vi "Actor Core.vi"(8 "error in":errorcluster, 11 "Nested in":refnum<class "Binary counter.lvclass">) -> (0 "error out":errorcluster, 3 "Actor out":refnum<class "Actor.lvclass">)   [LabVIEW 2020, in "Binary counter.lvlib" / "Binary counter.lvclass"]
doc: "(<B>Filename</B>: Actor Framework.lvlib:Actor.lvclass:Actor Core.vi)\n\nReceives messages to the actor, reacts to them, and initiates any error handling that may shut the actor down.\n\nDescendant classes may override this VI to append parallel tasks for the actor to complete while it handles messages. Overrides use the Call Parent Method node."
uses:
  Binary counter.lvclass
  C:/Program Files/National Instruments/LabVIEW 2020/vi.lib/ActorFramework/Actor/Actor.lvclass
  <vilib>/ActorFramework/Actor/Actor.lvclass
  Measurement_Binary/Measurement_Binary/Measurement_Binary.lvclass
  Binary counter.lvclass/Binary counter.ctl
  <vilib>/ActorFramework/Actor/Actor.lvclass/Actor.ctl
  <vilib>/ActorFramework/Message Enqueuer/Message Enqueuer.lvclass/Message Enqueuer.ctl
  Measurement_Binary/Measurement_Binary Messages/Start stop Msg/Start stop Msg.lvclass/Start stop Msg.ctl
  Measurement_Binary/Measurement_Binary Messages/Minimo Msg/Minimo Msg.lvclass/Minimo Msg.ctl
  Measurement_Binary/Measurement_Binary Messages/Maximo Msg/Maximo Msg.lvclass/Maximo Msg.ctl
  <vilib>/ActorFramework/Message Enqueuer/Init from Existing Queue.vi
  <vilib>/ActorFramework/Message Enqueuer/Enqueue.vi
  <vilib>/ActorFramework/Stop Msg/Stop Msg.lvclass
  C:/Program Files/National Instruments/LabVIEW 2020/vi.lib/ActorFramework/Message/Message.lvclass
  Measurement_Binary/Measurement_Binary Messages/Start stop Msg/Start stop Msg.lvclass
  Measurement_Binary/Measurement_Binary Messages/Minimo Msg/Minimo Msg.lvclass
  Measurement_Binary/Measurement_Binary Messages/Maximo Msg/Maximo Msg.lvclass
  <vilib>/ActorFramework/Message Priority Queue/Priority Enqueue.vi
  <vilib>/ActorFramework/Message Enqueuer/Message Enqueuer.lvclass
panel:
  out "Leds":bool[](array[boolean])
  in  "Máximo":u8
  in  "Mínimo":u8
  in  "Exit":bool
  in  "File Path":path
  in  "Save Format":u16(ring)
  in  "Save":bool
  in  "Stop":bool
  in  "Start":bool
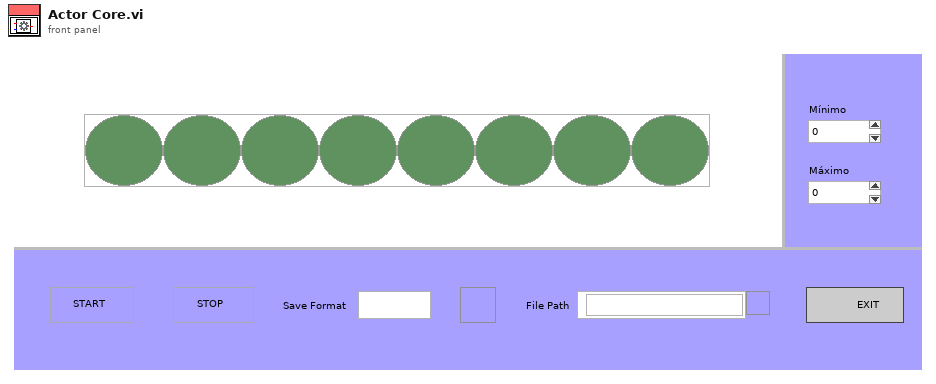
[diagram p1: front panel]
types:
  T1 = cluster{"Stop":refnum<user-event>, "Leds":refnum<user-event>}
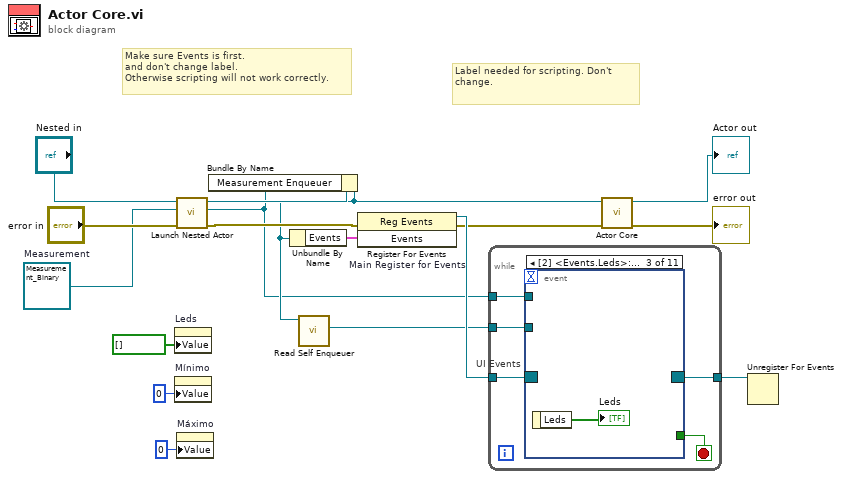
[diagram p0: block diagram]
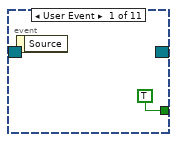
[diagram p2: hidden frame]
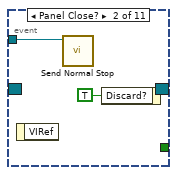
[diagram p3: hidden frame]
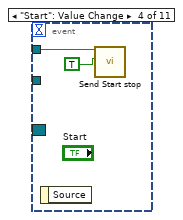
[diagram p4: hidden frame]
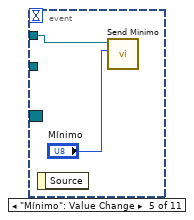
[diagram p5: hidden frame]
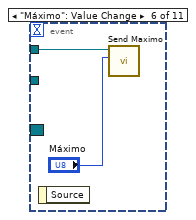
[diagram p6: hidden frame]
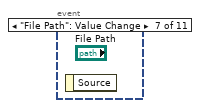
[diagram p7: hidden frame]
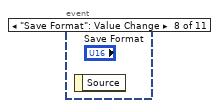
[diagram p8: hidden frame]
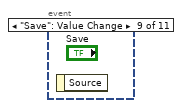
[diagram p9: hidden frame]
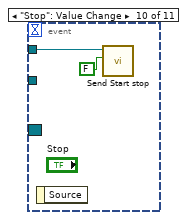
[diagram p10: hidden frame]
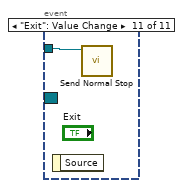
[diagram p11: hidden frame]
diagram:
  w6 = refnum<class "Measurement_Binary.lvclass"> refnum  # Measurement
  # "Label needed for scripting. Don't change."
  # "Make sure Events is first.\nand don't change label.\nOtherwise scripting will not work correctly."
  n1 = property on="Leds" class="Arr (strict)"("Value"=bool[] [] ("Leds")) -> ()  [unwired: 2 in, 2 out]
  n2 = property on="Mínimo" class="DigNum (strict)"("Value"=u8 0 ("Mínimo")) -> ()  [unwired: 2 in, 2 out]
  n3 = call <vilib>:"Launch Nested Actor.vi"("error in (no error)"="error in", "Nested Actor"=w6, "Caller Actor in"="Nested in") -> ("error out"=w7:errorcluster, "Nested Actor's Enqueuer"=w4:refnum<class "Message Enqueuer.lvclass">, "Caller Actor out"=w8:refnum<class "Binary counter.lvclass">)  [unwired: 6 in]
  n4 = property on="Máximo" class="DigNum (strict)"("Value"=u8 0 ("Máximo")) -> ()  [unwired: 2 in, 2 out]
  n5 = Bundle By Name(cluster=w8, "Measurement Enqueuer"=w4) -> (w5:refnum<class "Binary counter.lvclass">)
  n6 = Unbundle By Name(w5) -> ("Events"=w14:T1)
  n7 = call <vilib>:"Read Self Enqueuer.vi"("Actor"=w5) -> ("Self Enqueuer"=w12:refnum<class "Message Enqueuer.lvclass">)  [unwired: 10 in]
  n8 = register-events "Main Register for Events"(error in=w7, w14) -> (reference out=w15:refnum<event-registration>, error out=w11:errorcluster)  [unwired: 1 in]
  n9 = while {
    tunnel: w15 -> [w22]
    tunnel: [w20] -> w13
    tunnel: w12 -> [w19]
    tunnel: w4 -> [w18]
    stop <- w21 stop-if-true
    n10 = event "UI Events" shown="[2] <Events.Leds>: User Event" {
      selector: w22 -> [_ _ _ _ _ _ _ _ _ _ _]
      dyn-events: [_ _ _ _ _ _ _ _ _ _ _] -> w20
      timeout: _ -> [_ _ _ _ _ _ _ _ _ _ _]
      tunnel: [TRUE _ _ _ _ _ _ _ _ _ _] -> w21
      tunnel: w19 -> [_ w24 _ _ _ _ _ _ _ _ w35]
      tunnel: w18 -> [_ _ _ w28 w30 w32 _ _ _ w34 _]
      event User Event {
        n11 = event-data() -> ()  [unwired: 1 in, 1 out]
      }
      event Panel Close? {
        n12 = event-data() -> ()  [unwired: 1 in, 1 out]
        n13 = call <vilib>:"Send Normal Stop.vi"("Message Enqueuer"=w24) -> ()  [unwired: 10 in, 1 out]
        n14 = event-data("Discard?"=TRUE) -> ()  [unwired: 1 in, 1 out]
      }
      event User Event {
        n15 = event-data() -> ("Leds"=→"Leds":bool[])  [unwired: 1 in]
      }
      event "Start": Value Change {
        n16 = event-data() -> ()  [unwired: 1 in, 1 out]
        n17 = call "Send Start stop.vi"("Start/stop"=TRUE, "Message Enqueuer"=w28) -> ()  [unwired: 8 in, 2 out]
      }
      event "Mínimo": Value Change {
        n18 = event-data() -> ()  [unwired: 1 in, 1 out]
        n19 = call "Send Minimo.vi"("Minimo"="Mínimo", "Message Enqueuer"=w30) -> ()  [unwired: 8 in, 2 out]
      }
      event "Máximo": Value Change {
        n20 = event-data() -> ()  [unwired: 1 in, 1 out]
        n21 = call "Send Maximo.vi"("Maximo"="Máximo", "Message Enqueuer"=w32) -> ()  [unwired: 8 in, 2 out]
      }
      event "File Path": Value Change {
        n22 = event-data() -> ()  [unwired: 1 in, 1 out]
      }
      event "Save Format": Value Change {
        n23 = event-data() -> ()  [unwired: 1 in, 1 out]
      }
      event "Save": Value Change {
        n24 = event-data() -> ()  [unwired: 1 in, 1 out]
      }
      event "Stop": Value Change {
        n25 = event-data() -> ()  [unwired: 1 in, 1 out]
        n26 = call "Send Start stop.vi"("Start/stop"=FALSE, "Message Enqueuer"=w34) -> ()  [unwired: 8 in, 2 out]
      }
      event "Exit": Value Change {
        n27 = event-data() -> ()  [unwired: 1 in, 1 out]
        n28 = call <vilib>:"Send Normal Stop.vi"("Message Enqueuer"=w35) -> ()  [unwired: 10 in, 1 out]
      }
    }
  }
  n29 = call-parent "Actor Core.vi"("error in"=w11, "Actor in"=w5) -> ("error out"=→"error out":errorcluster, "Actor out"=→"Actor out":refnum<class "Actor.lvclass">)  [unwired: 8 in]
  n30 = Unregister For Events(event registration refnum=w13) -> ()  [unwired: 1 in, 1 out]
